vi "Resize_DiscardData_ARGB.vi"(8 "error in (no error)":errorcluster, 10 "New Image Size":T1, 11 "ARGB Image":refnum<data-value>) -> (0 "error out":errorcluster, 3 "ARGB Image (duplicate)":refnum<data-value>)   [LabVIEW 2020, in "g_ar_toolkit.lvlib"]
uses:
  Image Size Cluster.ctl
  OpenCV Interpolation Enum.ctl
  <vilib>/Utility/error.llb/Error Cluster From Error Code.vi
  g_ar_toolkit.lvlib
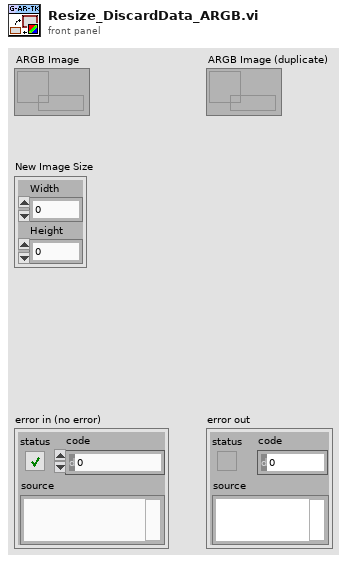
[diagram p1: front panel]
types:
  T1 = typedef "g_ar_toolkit.lvlib/Image Size Cluster.ctl" = cluster{"Width":u16, "Height":u16}
  T2 = typedef "g_ar_toolkit.lvlib/OpenCV Interpolation Enum.ctl" = enum16{"NEAREST", "LINEAR", "CUBIC", "AREA", "LANCZOS", "LINEAR_EXACT", "NEAREST_EXACT", "MAX"}
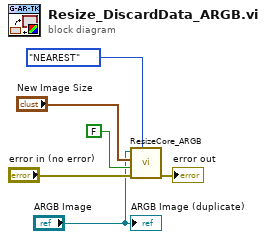
[diagram p0: block diagram]
diagram:
  n1 = call "ResizeCore_ARGB.vi"("OpenCV Interpolation Flag"=OpenCV_Interpolation_Enum."NEAREST", "error in (no error)"="error in (no error)", "Retain Data?"=FALSE, "ImageSize"="New Image Size", "ARGB Image"="ARGB Image") -> ("error out"=→"error out":errorcluster)  [unwired: 6 in]
  "ARGB Image (duplicate)" <- "ARGB Image"
